vi "Test1.vi"() -> ()   [LabVIEW 2024]
uses:
  C:/Program Files/National Instruments/LabVIEW 2024/WindowsFormsControlLibrary.dll
  Program Files/National Instruments/LabVIEW 2024/WindowsFormsControlLibrary.dll
panel:
  in  "UserControl1":refnum<k24>(container)
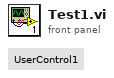
[diagram p1: front panel]
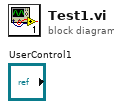
[diagram p0: block diagram]
diagram:
